vi "Th2829STRAT_RUN.vi"(8 "错误输入（无错误）":errorcluster, 11 "VISA资源名称":refnum<visa-resource-name>) -> (0 "error out":errorcluster, 2 "read buffer":string, 3 "read buffer 2":string, 5 "VISA资源名称 2":refnum<visa-resource-name>)   [LabVIEW 2018]
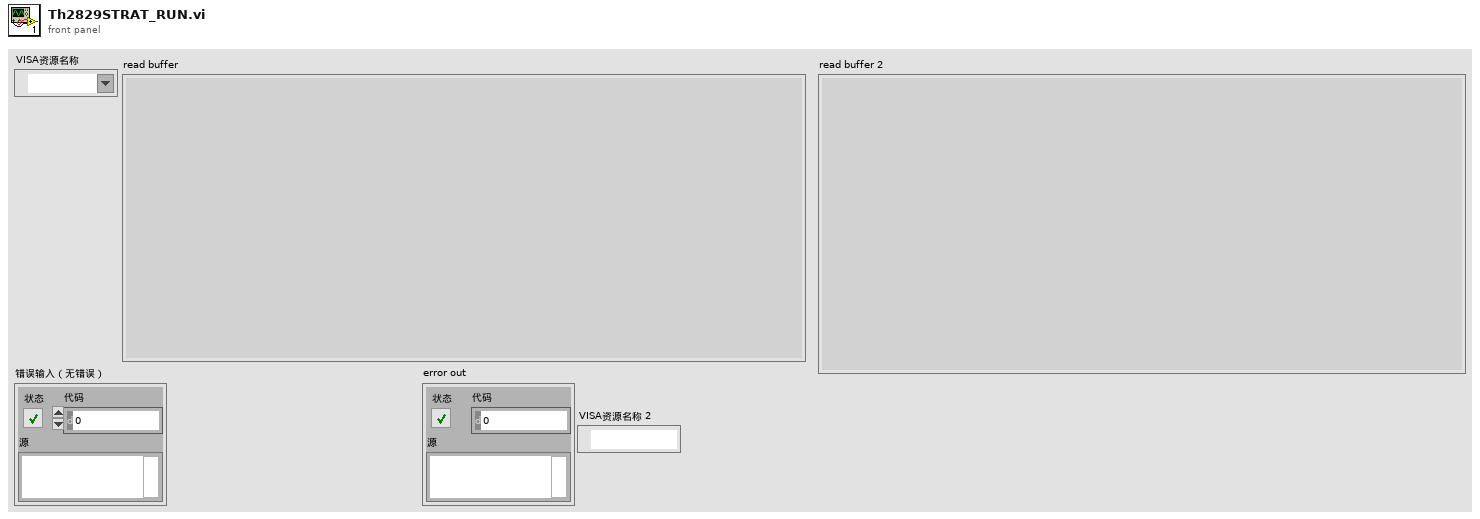
[diagram p1: front panel]
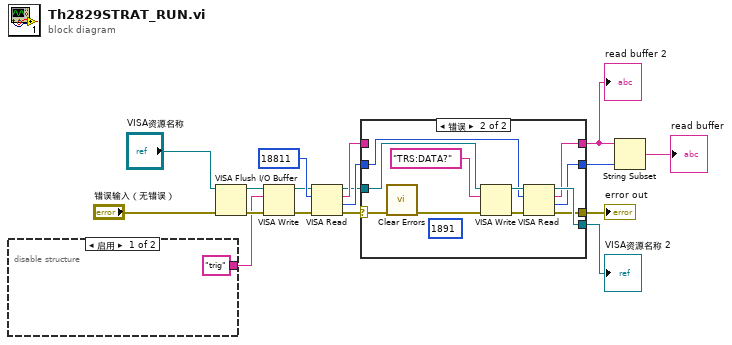
[diagram p0: block diagram]
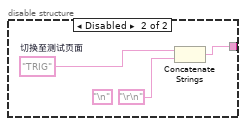
[diagram p2: hidden frame]
diagram:
  n1 = disable-structure shown="启用" {
    disable-tunnel: ["trig" ("write buffer") w20] -> w1
    frame Enabled {
    }
    frame Disabled {
      (unwired) "\n"
      w21 = "TRIG"  # 切换至测试页面
      n2 = Concatenate Strings(w21, "\r\n") -> (w20:string)
    }
  }
  n3 = VISA Flush I/O Buffer(VISA resource name="VISA资源名称", error in (no error)="错误输入（无错误）") -> (VISA resource name out=w17:refnum<visa-resource-name>, error out=w16:errorcluster)  [unwired: 1 in]
  n4 = VISA Write(VISA resource name=w17, write buffer=w1, error in (no error)=w16) -> (VISA resource name out=w9:refnum<visa-resource-name>, error out=w8:errorcluster)  [unwired: 1 out]
  n5 = VISA Read(VISA resource name=w9, byte count=u32 18811 ("字节总数"), error in (no error)=w8) -> (VISA resource name out=w12:refnum<visa-resource-name>, read buffer=w14:string, return count=w13:u32, error out=w11:errorcluster)
  n6 = case shown="错误" w11 {
    selector: w11 -> [w25 w32]
    tunnel: w12 -> [w24 w31]
    tunnel: [w24 w30] -> w2
    tunnel: [w25 w29] -> w7
    tunnel: [w22 w28] -> w5
    tunnel: [w23 w27] -> w4
    tunnel: w13 -> [w23 w26]
    tunnel: w14 -> [w22 _]
    frame No Error {
    }
    frame Error {
      (unwired) u32 1891 ("字节总数")
      n7 = call <vilib>:"Clear Errors.vi"("error in (no error)"=w32) -> ("error out"=w33:errorcluster)  [unwired: 5 in, 1 out]
      n8 = VISA Write(VISA resource name=w31, write buffer="TRS:DATA?", error in (no error)=w33) -> (VISA resource name out=w35:refnum<visa-resource-name>, error out=w36:errorcluster)  [unwired: 1 out]
      n9 = VISA Read(VISA resource name=w35, byte count=w26, error in (no error)=w36) -> (VISA resource name out=w30:refnum<visa-resource-name>, read buffer=w28:string, return count=w27:u32, error out=w29:errorcluster)
    }
  }
  "error out" <- w7
  "read buffer 2" <- w5
  "VISA资源名称 2" <- w2
  n10 = String Subset(string=w5, length (rest)=w4) -> (substring=→"read buffer":string)  [unwired: 1 in]
